vi "alarm sound.vi"(8 "error in (no error)":errorcluster, 11 "path":path=path "C:/Users/Public/Music/Sample Music/alert_siren.wav") -> (0 "error out":errorcluster)   [LabVIEW 2019]
uses:
  <vilib>/sound2/lvsound2.llb/Sampling Mode.ctl
  <vilib>/sound2/lvsound2.llb/Sound File Info (path).vi
  <vilib>/sound2/lvsound2.llb/Sound File Read Open.vi
  <vilib>/sound2/lvsound2.llb/Sound File Read (DBL).vi
  <vilib>/sound2/lvsound2.llb/Sound Output Write (DBL).vi
panel:
  in  "Number of Samples/Iteration":i32=2500
  in  "Device ID":u32
  in  "Stop":bool
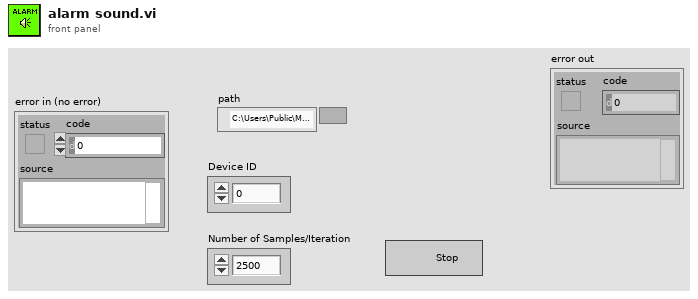
[diagram p1: front panel]
types:
  T1 = typedef "Sampling Mode.ctl" = i32
  T2 = typedef "Sound Data Format.ctl" = cluster{"sample rate (S/s)":dbl, "number of channels":i32, "bits per sample":i32}
  T3 = typedef "Sound File Refnum.ctl" = refnum<file>
  T4 = typedef "Sound Output Task ID.ctl" = u32
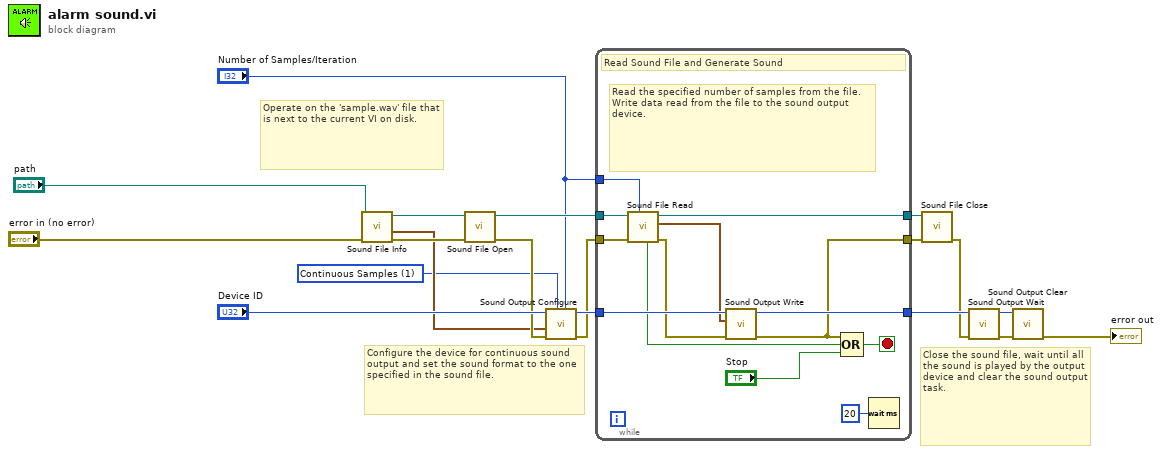
[diagram p0: block diagram]
diagram:
  w4 = T1 1 items=["Finite Samples", "Continuous Samples"] ("sample mode")
  # "Operate on the 'sample.wav' file that is next to the current VI on disk."
  # "Close the sound file, wait until all the sound is played by the output device and clear the sound output task."
  # "Configure the device for continuous sound output and set the sound format to the one specified in the sound file."
  n1 = call-poly <vilib>:"Sound File Info.vi"("error in (no error)"="error in (no error)", "path"="path") -> ("error out"=w14:errorcluster, "sound format"=w6:T2, "path out"=w7:path)  [unwired: 6 in, 1 out]
  n2 = call-poly <vilib>:"Sound File Open.vi"("error in (no error)"=w14, "path"=w7) -> ("error out"=w13:errorcluster, "sound file refnum"=w15:T3)  [unwired: 8 in]
  n3 = call <vilib>:"Sound Output Configure.vi"("number of samples/ch"="Number of Samples/Iteration", "sample mode"=w4, "error in (no error)"=w13, "sound format"=w6, "device ID"="Device ID") -> ("error out"=w12:errorcluster, "task ID"=w19:T4)  [unwired: 5 in]
  n4 = while {
    tunnel: "Number of Samples/Iteration" -> [w23]
    tunnel: w15 -> [w30]
    tunnel: [w29] -> w17
    tunnel: w12 -> [w31]
    tunnel: [w22] -> w16
    tunnel: w19 -> [w28]
    tunnel: [w32] -> w10
    stop <- w24 stop-if-true
    # "Read the specified number of samples from the file. Write data read from the file to the sound output device."
    # "Read Sound File and Generate Sound"
    n5 = call-poly <vilib>:"Sound File Read.vi"("number of samples/ch (-1: all)"=w23, "error in (no error)"=w31, "sound file refnum"=w30) -> ("error out"=w27:errorcluster, "data"=w21:waveform(dbl)[], "sound file refnum out"=w29:T3, "end of file?"=w25:bool)  [unwired: 4 in, 1 out]
    n6 = call-poly <vilib>:"Sound Output Write.vi"("error in (no error)"=w27, "data"=w21, "task ID"=w28) -> ("error out"=w22:errorcluster, "task ID out"=w32:T4)  [unwired: 7 in]
    n7 = Compound Arithmetic op=OR(w22, w25, "Stop") -> (w24:bool)
    n8 = Wait (ms)(milliseconds to wait=u32 20) -> ()  [unwired: 1 out]
  }
  n9 = call <vilib>:"Sound File Close.vi"("error in (no error)"=w16, "sound file refnum"=w17) -> ("error out"=w9:errorcluster)  [unwired: 9 in]
  n10 = call <vilib>:"Sound Output Wait.vi"("error in (no error)"=w9, "task ID"=w10) -> ("error out"=w8:errorcluster, "task ID out"=w11:T4)  [unwired: 8 in]
  n11 = call <vilib>:"Sound Output Clear.vi"("error in (no error)"=w8, "task ID"=w11) -> ("error out"=→"error out":errorcluster)  [unwired: 9 in]
